vi "DESTROY UE.vi"(8 "error in (no error)":errorcluster, 11 "DATABASE_MANEJO in":refnum<class "DATABASE_MANEJO.lvclass">) -> (0 "error out":errorcluster, 3 "DATABASE_MANEJO out":refnum<class "DATABASE_MANEJO.lvclass">)   [LabVIEW 2019, in "DATABASE_MANEJO.lvlib" / "DATABASE_MANEJO.lvclass"]
uses:
  DATABASE_MANEJO.lvclass
  DATABASE_MANEJO.lvclass/DATABASE_MANEJO.ctl
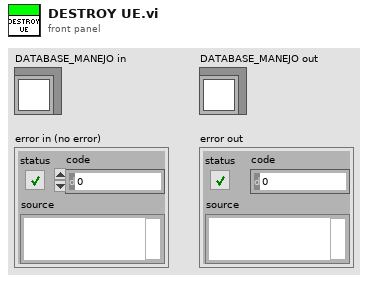
[diagram p1: front panel]
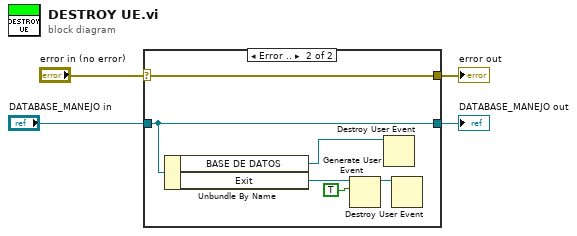
[diagram p0: block diagram]
diagram:
  n1 = case shown="Error .." "error in (no error)" {
    selector: "error in (no error)" -> [w6 w7]
    tunnel: [w6 w7] -> w2
    tunnel: [w5 w8] -> w4
    tunnel: "DATABASE_MANEJO in" -> [w5 w8]
    frame No Error {
    }
    frame Error {
      n2 = Unbundle By Name(w8) -> ("BASE DE DATOS"=w9:refnum<user-event>, "Exit"=w12:refnum<user-event>)
      n3 = Generate User Event(user event=w12, event data cluster=TRUE ("event data")) -> (user event out=w10:refnum<user-event>)  [unwired: 2 in, 1 out]
      n4 = Destroy User Event(user event=w9) -> ()  [unwired: 1 in, 1 out]
      n5 = Destroy User Event(user event=w10) -> ()  [unwired: 1 in, 1 out]
    }
  }
  "DATABASE_MANEJO out" <- w4
  "error out" <- w2
